vi "Build_Request.vi"(8 "error in (no error)":errorcluster, 10 "Application":T1, 11 "OAuth in":refnum<class "OAuth.lvclass">) -> (0 "error out":errorcluster, 3 "OAuth out":refnum<class "OAuth.lvclass">)   [LabVIEW 2016, in "OAuth.lvclass"]
uses:
  OAuth.lvclass
  scope_needed.ctl
  OAuth.lvclass/OAuth.ctl
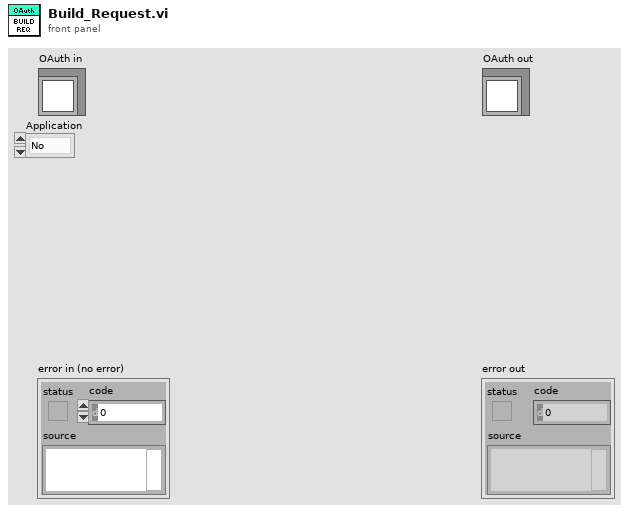
[diagram p1: front panel]
types:
  T1 = typedef "scope_needed.ctl" = enum16{"No", "Yes"}
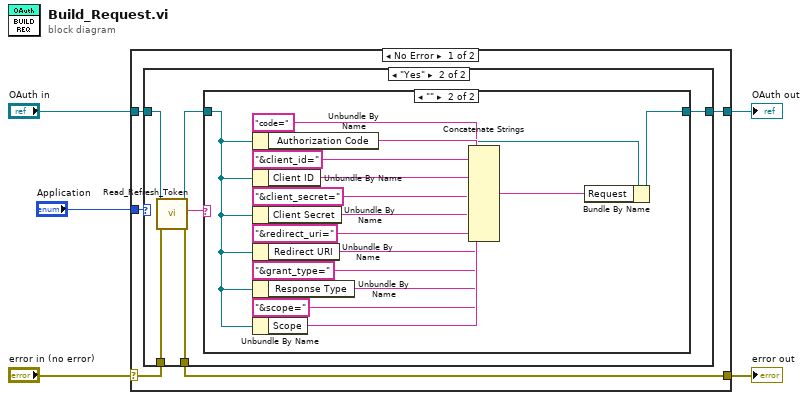
[diagram p0: block diagram]
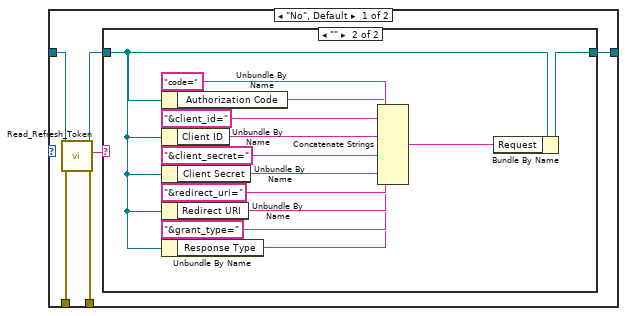
[diagram p2: hidden frame]
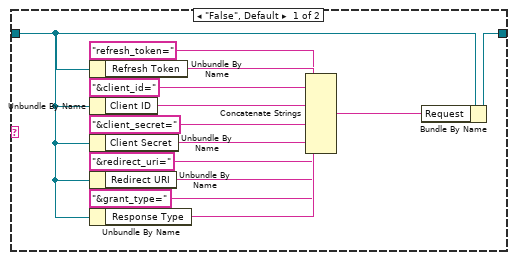
[diagram p3: hidden frame]
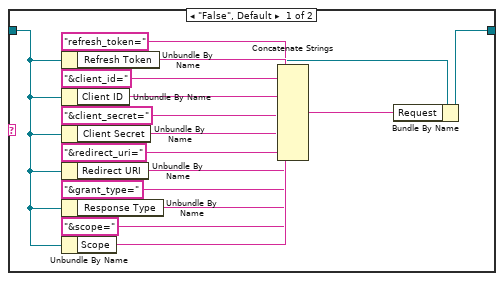
[diagram p4: hidden frame]
diagram:
  n1 = case shown="No Error" "error in (no error)" {
    selector: "error in (no error)" -> [w8 w80]
    tunnel: [w7 w80] -> w4
    tunnel: "OAuth in" -> [w9 w79]
    tunnel: "Application" -> [w10 _]
    tunnel: [w6 w79] -> w1
    frame No Error {
      n2 = case shown="\"Yes\"" w10 {
        tunnel: w9 -> [w15 w45]
        tunnel: w8 -> [w13 w48]
        tunnel: [w12 w47] -> w7
        tunnel: [w11 w43] -> w6
        frame "No", Default {
          n3 = call-dynamic "Read_Refresh_Token.vi"("error in (no error)"=w13, "OAuth in"=w15) -> ("error out"=w12:errorcluster, "String"=w16:string, "OAuth out"=w14:refnum<class "OAuth.lvclass">)  [unwired: 7 in]
          n4 = case shown="\"\"" w16 {
            tunnel: w14 -> [w18 w31]
            tunnel: [w17 w30] -> w11
            frame "False", Default {
              n5 = Unbundle By Name(w18) -> ("Refresh Token"=w21:string)
              n6 = Unbundle By Name(w18) -> ("Client ID"=w23:string)
              n7 = Unbundle By Name(w18) -> ("Client Secret"=w25:string)
              n8 = Unbundle By Name(w18) -> ("Redirect URI"=w27:string)
              n9 = Unbundle By Name(w18) -> ("Response Type"=w29:string)
              n10 = Concatenate Strings("refresh_token=", w21, "&client_id=", w23, "&client_secret=", w25, "&redirect_uri=", w27, "&grant_type=", w29) -> (w19:string)
              n11 = Bundle By Name(cluster=w18, "Request"=w19) -> (w17:refnum<class "OAuth.lvclass">)
            }
            frame "" {
              n12 = Unbundle By Name(w31) -> ("Authorization Code"=w40:string)
              n13 = Unbundle By Name(w31) -> ("Client ID"=w38:string)
              n14 = Unbundle By Name(w31) -> ("Client Secret"=w36:string)
              n15 = Unbundle By Name(w31) -> ("Redirect URI"=w34:string)
              n16 = Unbundle By Name(w31) -> ("Response Type"=w32:string)
              n17 = Concatenate Strings("code=", w40, "&client_id=", w38, "&client_secret=", w36, "&redirect_uri=", w34, "&grant_type=", w32) -> (w42:string)
              n18 = Bundle By Name(cluster=w31, "Request"=w42) -> (w30:refnum<class "OAuth.lvclass">)
            }
          }
        }
        frame "Yes" {
          n19 = call-dynamic "Read_Refresh_Token.vi"("error in (no error)"=w48, "OAuth in"=w45) -> ("error out"=w47:errorcluster, "String"=w46:string, "OAuth out"=w44:refnum<class "OAuth.lvclass">)  [unwired: 7 in]
          n20 = case shown="\"\"" w46 {
            tunnel: w44 -> [w50 w65]
            tunnel: [w49 w64] -> w43
            frame "False", Default {
              n21 = Unbundle By Name(w50) -> ("Refresh Token"=w52:string)
              n22 = Unbundle By Name(w50) -> ("Client ID"=w55:string)
              n23 = Unbundle By Name(w50) -> ("Client Secret"=w57:string)
              n24 = Unbundle By Name(w50) -> ("Redirect URI"=w59:string)
              n25 = Unbundle By Name(w50) -> ("Response Type"=w61:string)
              n26 = Unbundle By Name(w50) -> ("Scope"=w63:string)
              n27 = Concatenate Strings("refresh_token=", w52, "&client_id=", w55, "&client_secret=", w57, "&redirect_uri=", w59, "&grant_type=", w61, "&scope=", w63) -> (w54:string)
              n28 = Bundle By Name(cluster=w50, "Request"=w54) -> (w49:refnum<class "OAuth.lvclass">)
            }
            frame "" {
              n29 = Unbundle By Name(w65) -> ("Authorization Code"=w67:string)
              n30 = Unbundle By Name(w65) -> ("Client ID"=w70:string)
              n31 = Unbundle By Name(w65) -> ("Client Secret"=w72:string)
              n32 = Unbundle By Name(w65) -> ("Redirect URI"=w74:string)
              n33 = Unbundle By Name(w65) -> ("Response Type"=w76:string)
              n34 = Unbundle By Name(w65) -> ("Scope"=w78:string)
              n35 = Concatenate Strings("code=", w67, "&client_id=", w70, "&client_secret=", w72, "&redirect_uri=", w74, "&grant_type=", w76, "&scope=", w78) -> (w69:string)
              n36 = Bundle By Name(cluster=w65, "Request"=w69) -> (w64:refnum<class "OAuth.lvclass">)
            }
          }
        }
      }
    }
    frame Error {
    }
  }
  "error out" <- w4
  "OAuth out" <- w1
